vi "Test line.vi"() -> ()   [LabVIEW 2015]
panel:
  in  "Line":T1={"Point 1"={"X"=50.0, "Y"=50.0}, "Point 2"={"X"=150.0, "Y"=150.0}}
  out "Image":T2(plugin-control)
  out "error out":errorcluster
  in  "error in (no error)":errorcluster
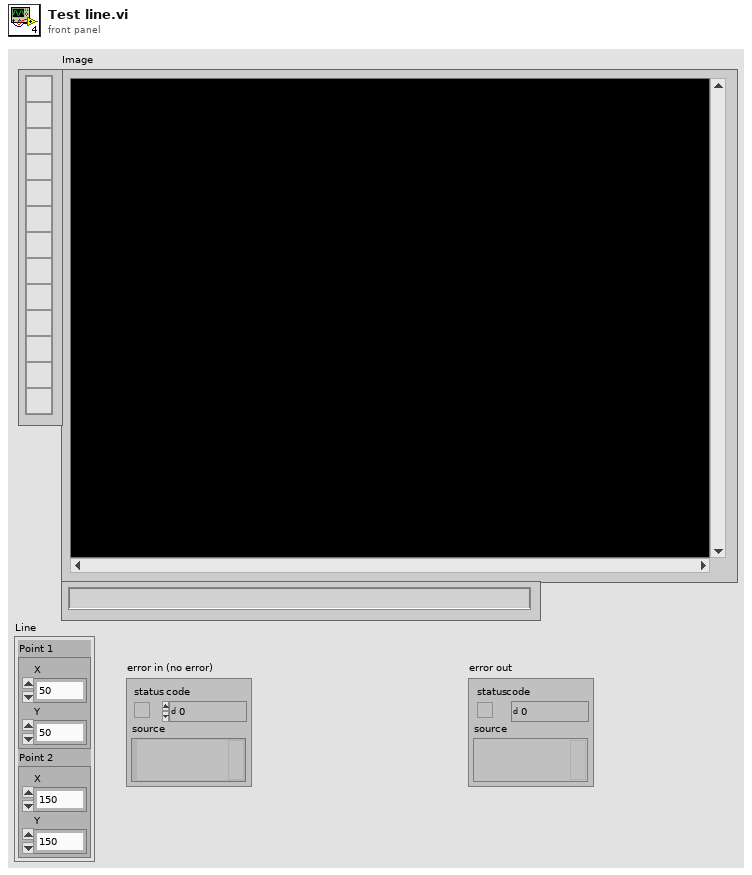
[diagram p1: front panel]
types:
  T1 = cluster{"Point 1":cluster{"X":sgl, "Y":sgl}, "Point 2":cluster{"X":sgl, "Y":sgl}}
  T2 = typedef "IMAQ Image.ctl" = refnum<image>
  T3 = cluster{"Global Rectangle":i32[], "Contours":cluster{"Contour Type":u32, "ROI Type":u32, "Points":i32[]}[]}
  T4 = typedef "IMAQ Point" = cluster{"X":sgl, "Y":sgl}
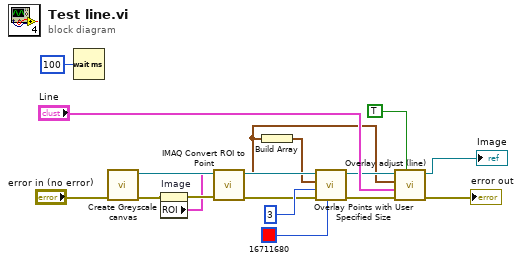
[diagram p0: block diagram]
diagram:
  n1 = Wait (ms)(milliseconds to wait=u32 100) -> ()  [unwired: 1 out]
  n2 = call "Create Greyscale canvas.vi"("error in (no error)"="error in (no error)") -> ("error out"=w7:errorcluster, "Image"=w13:T2)  [unwired: 9 in]
  n3 = property on="Image" class="ImageControl"(error in=w7) -> (error out=w6:errorcluster, "ROI"=w4:T3)  [unwired: 1 in, 1 out]
  n4 = call "IMAQ Convert ROI to Point"("error in (no error)"=w6, "ROI Descriptor"=w4) -> ("error out"=w5:errorcluster, "Point"=w3:T4)  [unwired: 7 in]
  n5 = Build Array(w3) -> (w11:T4[])
  n6 = call "Overlay Points with User Specified Size.vi"("Color"=u32 16711680, "error in"=w5, "Point Diameter (5)"=u32 3, "Points"=w11, "Image In"=w13) -> ("error out"=w14:errorcluster, "Image Out"=w12:T2)  [unwired: 5 in]
  n7 = call "Overlay adjust (line).vi"("Enable overlay?"=TRUE, "error in (no error)"=w14, "Line"="Line", "Mouse release point"=w3, "Image"=w12) -> ("error out"=→"error out":errorcluster, "Image Out"=→"Image":T2)  [unwired: 4 in, 1 out]
